vi "System Explorer - Add extra pages to System Explorer library.vi"(8 "error in (no error)":errorcluster, 9 "Extra Page Names":string[](array[string]), 10 "Project Root":path, 11 "ProjectItem in":refnum<vi>) -> (0 "error out":errorcluster, 2 "Extra Page VIs":path[](array[path]), 3 "ProjectItem out":refnum<vi>)   [LabVIEW 2020, in "NIVS_Consolidated_CDW_MetaDataObj.lvclass"]
doc: "Create an addition folder under the ProjectItem and add all created extra pages to this folder."
uses:
  NIVS_Consolidated_CDW_MetaDataObj.lvclass
  CD System Explorer lvlib.ctl
  Add Item - Type.ctl
  CD System Explorer lvlib.vi
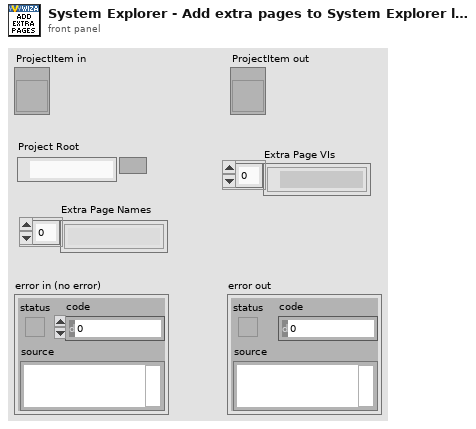
[diagram p1: front panel]
types:
  T1 = typedef "NIVS_Consolidated_CDW_MetaDataObj.lvclass/CD System Explorer lvlib.ctl" = enum16{"LibraryFileName", "LibraryFolderName", "System Explorer.FolderName", "System Explorer.Dynamically Called.FolderName", "System Explorer.Dynamically Called.Extra Pages.FolderName", "System Explorer.Dynamically Called.Extra Pages.TemplatePathAndName", "System Explorer.Dynamically Called.Main Page.VIName", "System Explorer.Dynamically Called.Main Page.TemplatePathAndName", "System Explorer.Dynamically Called.Initialization VI.VIName", "System Explorer.Dynamically Called.Initialization VI.TemplatePathAndName", "System Explorer.SubVI.FolderName", "System Explorer.Types.FolderName", "System Explorer.ActionVIOnCompile.VIName", "System Explorer.ExportConfigRTM.VIName", "System Explorer.PPL.ExportConfigRTM.VIName", "System Explorer.LoadHelpFile.VIName", "System Explorer.PPL.LoadHelpFile.VIName", "System Explorer.SetRTDriverVIsFilePaths.VIName", "System Explorer.ClearRTDriverVIs.VIName"}
  T2 = typedef "NIVS_Consolidated_CDW_MetaDataObj.lvclass/Add Item - Type.ctl" = string
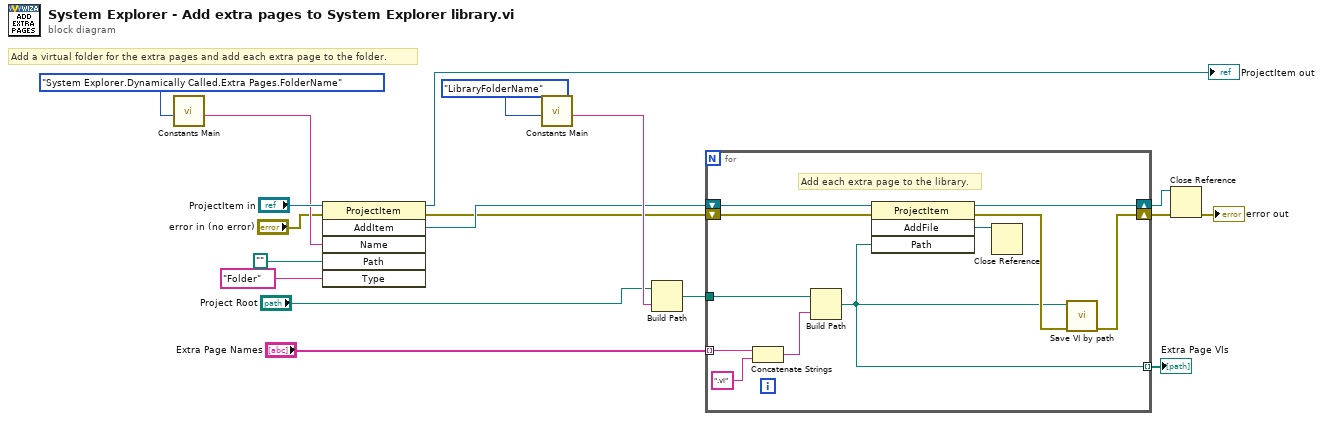
[diagram p0: block diagram]
diagram:
  # "Add a virtual folder for the extra pages and add each extra page to the folder."
  n1 = call-poly "Constants Main.vi"("Action"=CD_System_Explorer_lvlib."System Explorer.Dynamically Called.Extra Pages.FolderName") -> ("Output"=w13:string)  [unwired: 10 in]
  n2 = invoke class="ProjectItem" method="AddItem"(reference="ProjectItem in", error in="error in (no error)", "Name"=w13, "Path"=path "", "Type"=T2 "Folder" ("Add Item - Type")) -> (reference out=→"ProjectItem out":refnum<vi>, error out=w4:errorcluster, "AddItem"=w8:refnum<vi>)  [unwired: 1 in, 3 out]
  n3 = call-poly "Constants Main.vi"("Action"=CD_System_Explorer_lvlib."LibraryFolderName") -> ("Output"=w10:string)  [unwired: 10 in]
  n4 = Build Path(base path="Project Root", name or relative path=w10) -> (appended path=w9:path)
  n5 = for {
    shift-right: [w27] -> w6
    shift-left: w8 -> [w29]
    shift-right: [w22] -> w7
    shift-left: w4 -> [w28]
    tunnel: w9 -> [w24]
    tunnel: "Extra Page Names" -> [w21] mode=indexing
    tunnel: [w20] -> w1 mode=indexing
    # "Add each extra page to the library."
    n6 = Concatenate Strings(w21, ".vi") -> (w25:string)
    n7 = Build Path(base path=w24, name or relative path=w25) -> (appended path=w20:path)
    n8 = invoke class="ProjectItem" method="AddFile"(reference=w29, error in=w28, "Path"=w20) -> (reference out=w27:refnum<vi>, error out=w23:errorcluster, "AddFile"=w19:refnum<vi>)  [unwired: 1 in, 1 out]
    n9 = Close Reference(reference=w19) -> ()  [unwired: 1 in, 1 out]
    n10 = call "Save VI by path.vi"("error in (no error)"=w23, "VI path"=w20) -> ("error out"=w22:errorcluster)  [unwired: 9 in]
  }
  "Extra Page VIs" <- w1
  n11 = Close Reference(reference=w6, error in (no error)=w7) -> (error out=→"error out":errorcluster)
